vi "Background Loop Step.vi"(8 "error in (no error)":errorcluster, 10 "Action":T1, 11 "Instrument Driver in":refnum<class "Instrument Driver.lvclass">) -> (0 "error out":errorcluster, 1 "Next step delay":i32, 2 "Action out":T1, 3 "Instrument Driver out":refnum<class "Instrument Driver.lvclass">, 4 "Result":refnum<class "Acquired Result.lvclass">)   [LabVIEW 2021, in "Instrument Driver.lvclass"]
uses:
  Instrument Driver.lvclass
  LabActor/Worker/Background Loop Action.ctl
  Instrument Driver.lvclass/Instrument Driver.ctl
  Results/Acquired Result/Acquired Result.lvclass
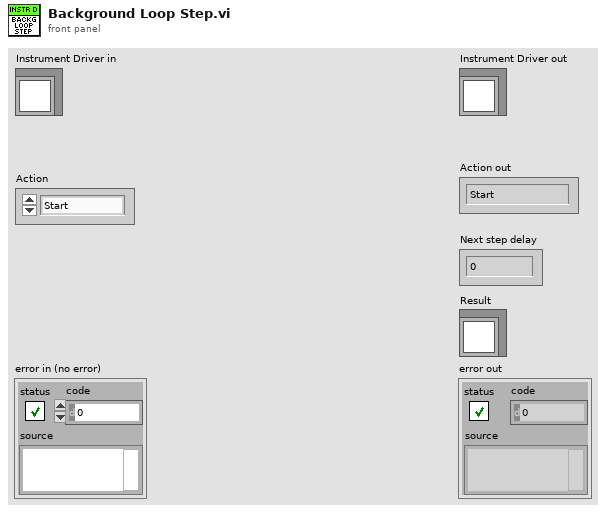
[diagram p1: front panel]
types:
  T1 = typedef "Background Loop Action.ctl" = enum16{"Start", "Continue", "Stop"}
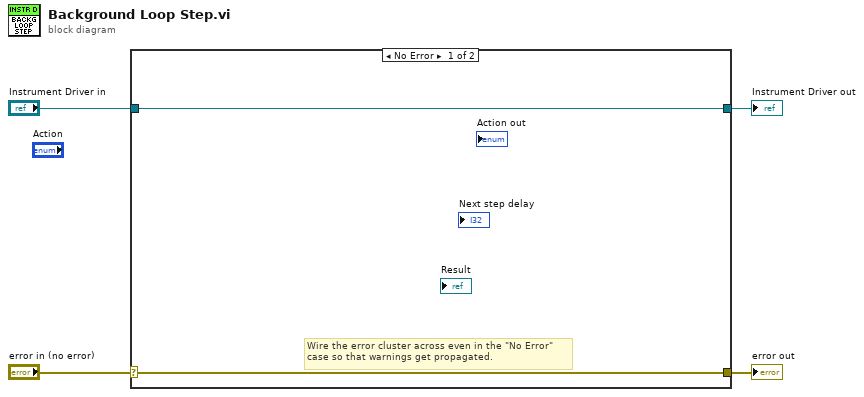
[diagram p0: block diagram]
diagram:
  n1 = case shown="No Error" "error in (no error)" {
    selector: "error in (no error)" -> [w5 w8]
    tunnel: [w5 w8] -> w3
    tunnel: [w6 w7] -> w1
    tunnel: "Instrument Driver in" -> [w6 w7]
    frame No Error {
      # "Wire the error cluster across even in the \"No Error\"\ncase so that warnings get propagated."
    }
    frame Error {
    }
  }
  "error out" <- w3
  "Instrument Driver out" <- w1
